vi "GetIoState.vi"(10 "Ftp":refnum<k24>, 11 "error in":errorcluster) -> (2 "IO States":T1(array[cluster]), 3 "error out":errorcluster)   [LabVIEW 2011, in "UnderAutomation.Fanuc.lvlib"]
uses:
  UnderAutomation.Fanuc.lvlib
  C:/Users/fg/Documents/Fanuc.vi/LabVIEW_2024/UnderAutomation.Fanuc/lib/UnderAutomation.Fanuc.dll
  LabVIEW_2024/UnderAutomation.Fanuc/lib/UnderAutomation.Fanuc.dll
panel:
  out "Port":i32(ring) items=["DIN", "DOUT", "UI", "UO", "SI", "SO", "RI", "RO", "FLG"]
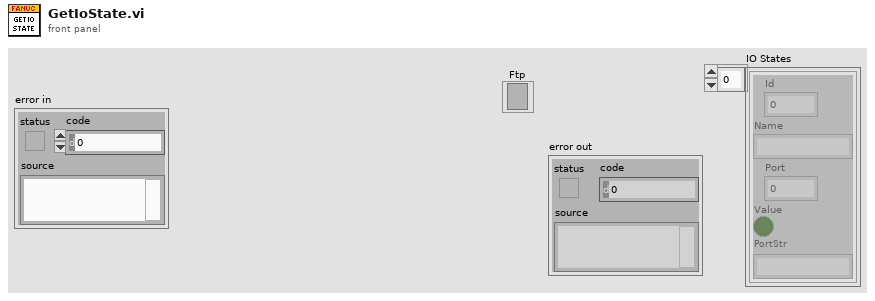
[diagram p1: front panel]
types:
  T1 = cluster{"Id":i32, "Name":string, "Port":i32, "Value":bool, "PortStr":string}[]
  T2 = cluster{"Id":i32, "Name":string, "Port":i32, "Value":bool, "RingText.Text":string}
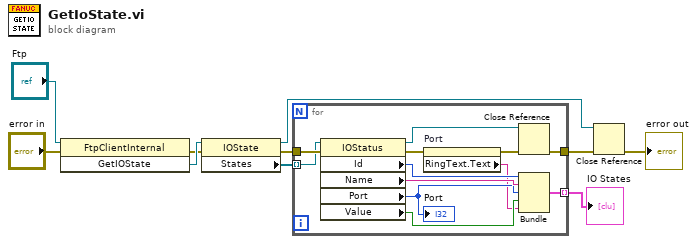
[diagram p0: block diagram]
diagram:
  n1 = invoke class="FtpClientInternal" method="GetIOState"(reference="Ftp", error in="error in") -> (error out=w7:errorcluster, "GetIOState"=w8:refnum<k24>)  [unwired: 1 in, 1 out]
  n2 = property class="IOState"(reference=w8, error in=w7) -> (reference out=w1:refnum<k24>, error out=w5:errorcluster, "States"=w6:refnum<k24>[])
  n3 = for {
    tunnel: w5 -> [w22]
    tunnel: [w11] -> w3
    tunnel: w6 -> [w21] mode=indexing
    tunnel: [w19] -> w4 mode=indexing
    n4 = property class="IOStatus"(reference=w21, error in=w22) -> (reference out=w13:refnum<k24>, error out=w14:errorcluster, "Id"=w20:i32, "Name"=w18:string, "Port"=w16:i32, "Value"=w17:bool)
    "Port" <- w16
    n5 = property on="Port" class="Ring (strict)"(error in=w14) -> (error out=w12:errorcluster, "RingText.Text"=w15:string)  [unwired: 1 in, 1 out]
    n6 = Close Reference(reference=w13, error in (no error)=w12) -> (error out=w11:errorcluster)
    n7 = Bundle("Id"=w20, "Name"=w18, "Port"=w16, "Value"=w17, "RingText.Text"=w15) -> (w19:T2)  [unwired: 1 in]
  }
  "IO States" <- w4
  n8 = Close Reference(reference=w1, error in (no error)=w3) -> (error out=→"error out":errorcluster)
